vi "channel_agent_forward.vi"() -> ()   [LabVIEW 2017]
doc: "Illustrates how to request agent forwarding on a channel."
uses:
  libssh2/libssh2_session_handshake_tcp.vi
  libssh2/libssh2_init_default.vi
  libssh2/libssh2_session_init_ex.vi
  <vilib>/Utility/tcp.llb/TCP Get Raw Net Object.vi
  libssh2/libssh2_session_handshake_socket.vi
  libssh2/libssh2_userauth_password_ex.vi
  libssh2/libssh2_channel_open_ex.vi
  libssh2/libssh2_channel_process_startup.vi
  libssh2/libssh2_channel_read_ex.vi
  libssh2/libssh2.lvlib
panel:
  in  "password":string
  in  "username":string
  in  "hostname":string="localhost"
  out "SSH_AUTH_SOCK":string
  out "error out":errorcluster
  # "When everything is right, then this variable is set."
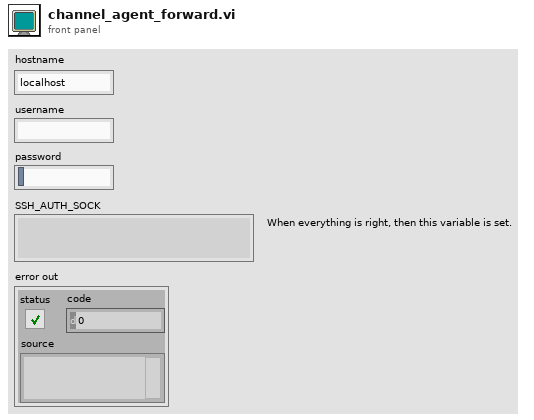
[diagram p1: front panel]
types:
  T1 = typedef "libssh2.lvlib/Session Refnum.ctl" = refnum<k1>
  T2 = typedef "libssh2.lvlib/Channel Refnum.ctl" = refnum<k1>
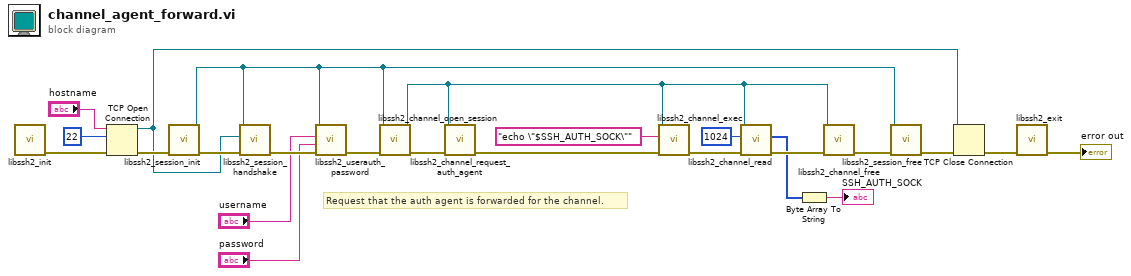
[diagram p0: block diagram]
diagram:
  # "Request that the auth agent is forwarded for the channel."
  n1 = call-poly "libssh2_init.vi"() -> ("error out"=w23:errorcluster)  [unwired: 11 in]
  n2 = TCP Open Connection(address="hostname", remote port or service name=u16 22, error in (no error)=w23) -> (connection ID=w6:refnum<k5>, error out=w13:errorcluster)  [unwired: 2 in]
  n3 = call "libssh2_session_init.vi"("error in (no error)"=w13) -> ("error out"=w10:errorcluster, "session"=w3:T1)  [unwired: 9 in]
  n4 = call-poly "libssh2_session_handshake.vi"("error in (no error)"=w10, "tcp connection"=w6, "session"=w3) -> ("error out"=w8:errorcluster)  [unwired: 8 in]
  n5 = call "libssh2_userauth_password.vi"("error in (no error)"=w8, "password"="password", "username"="username", "session"=w3) -> ("error out"=w1:errorcluster)  [unwired: 7 in]
  n6 = call "libssh2_channel_open_session.vi"("error in (no error)"=w1, "session"=w3) -> ("error out"=w22:errorcluster, "channel"=w17:T2)  [unwired: 8 in]
  n7 = call "libssh2_channel_request_auth_agent.vi"("error in (no error)"=w22, "channel"=w17) -> ("error out"=w21:errorcluster)  [unwired: 9 in]
  n8 = call "libssh2_channel_exec.vi"("error in (no error)"=w21, "command"="echo \"$SSH_AUTH_SOCK\"", "channel"=w17) -> ("error out"=w20:errorcluster)  [unwired: 8 in]
  n9 = call "libssh2_channel_read.vi"("error in (no error)"=w20, "buffer length"=1024, "channel"=w17) -> ("error out"=w18:errorcluster, "buffer"=w15:u8[])  [unwired: 7 in]
  n10 = Byte Array To String(unsigned byte array=w15) -> (string=→"SSH_AUTH_SOCK":string)
  n11 = call "libssh2_channel_free.vi"("error in (no error)"=w18, "channel"=w17) -> ("error out"=w2:errorcluster)  [unwired: 9 in]
  n12 = call "libssh2_session_free.vi"("error in (no error)"=w2, "session"=w3) -> ("error out"=w9:errorcluster)  [unwired: 9 in]
  n13 = TCP Close Connection(connection ID=w6, error in (no error)=w9) -> (error out=w7:errorcluster)  [unwired: 1 in, 1 out]
  n14 = call "libssh2_exit.vi"("error in (no error)"=w7) -> ("error out"=→"error out":errorcluster)  [unwired: 10 in]
